vi "Read Chamber Data.vi"(8 "error in (no error)":errorcluster, 11 "Chamber Controller in":refnum<class "Chamber Controller.lvclass">) -> (0 "error out":errorcluster, 3 "Chamber Controller out":refnum<class "Chamber Controller.lvclass">)   [LabVIEW 2020, in "Chamber Controller.lvlib" / "Chamber Controller.lvclass"]
uses:
  Chamber Controller.lvclass
  C:/Program Files (x86)/National Instruments/LabVIEW 2020/vi.lib/ActorFramework/Actor/Actor.lvclass
  <vilib>/ActorFramework/Actor/Actor.lvclass/Actor.ctl
  Chamber Controller.lvclass/Chamber Controller.ctl
  Chamber Controller Interface/Chamber Controller Interface Messages/Report Chamber Data Msg/Report Chamber Data Msg.lvclass/Report Chamber Data Msg.ctl
  <vilib>/ActorFramework/Message Enqueuer/Message Enqueuer.lvclass/Message Enqueuer.ctl
  <vilib>/ActorFramework/Message Enqueuer/Enqueue.vi
  Chamber Controller Interface/Chamber Controller Interface Messages/Report Chamber Data Msg/Report Chamber Data Msg.lvclass
  C:/Program Files (x86)/National Instruments/LabVIEW 2020/vi.lib/ActorFramework/Message/Message.lvclass
  <vilib>/ActorFramework/Message Priority Queue/Priority Enqueue.vi
  _Abstract Classes/Abstract Chamber/Abstract Chamber.lvclass
  <vilib>/ActorFramework/Actor/Actor.lvclass
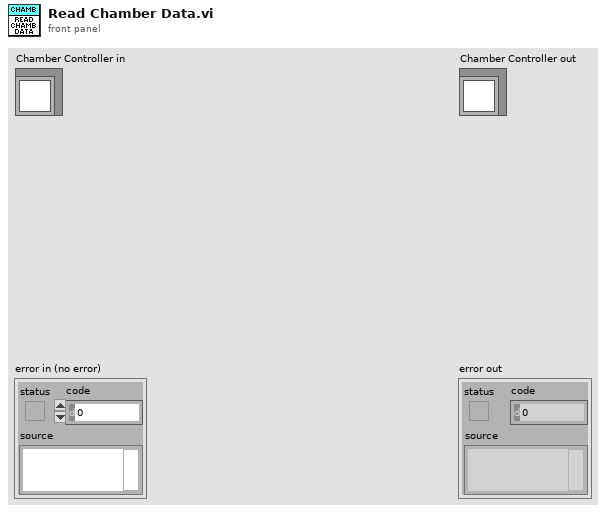
[diagram p1: front panel]
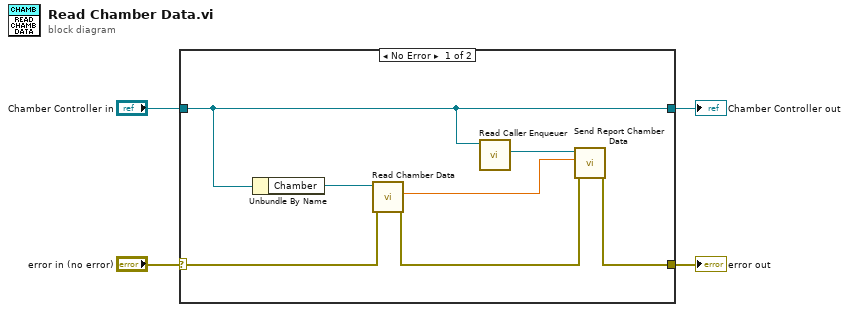
[diagram p0: block diagram]
diagram:
  n1 = case shown="No Error" "error in (no error)" {
    selector: "error in (no error)" -> [w10 w13]
    tunnel: [w5 w13] -> w3
    tunnel: [w9 w12] -> w1
    tunnel: "Chamber Controller in" -> [w9 w12]
    frame No Error {
      n2 = Unbundle By Name(w9) -> ("Chamber"=w11:refnum<class "Abstract Chamber.lvclass">)
      n3 = call-dynamic "Read Chamber Data.vi"("error in (no error)"=w10, "Abstract Chamber in"=w11) -> ("error out"=w6:errorcluster, "Temp (C)"=w7:dbl)  [unwired: 7 in, 1 out]
      n4 = call <vilib>:"Read Caller Enqueuer.vi"("Actor"=w9) -> ("Caller Enqueuer"=w8:refnum<class "Message Enqueuer.lvclass">)  [unwired: 10 in]
      n5 = call "Send Report Chamber Data.vi"("error in (no error)"=w6, "Temp (C)"=w7, "Message Enqueuer"=w8) -> ("error out"=w5:errorcluster)  [unwired: 7 in, 1 out]
    }
    frame Error {
    }
  }
  "error out" <- w3
  "Chamber Controller out" <- w1
